vi "MotorsGoToLimits.vi"(11 "output cluster":T1) -> (0 "error out":errorcluster)   [LabVIEW 2015]
uses:
  Controls/LP Motor Thread Data.ctl
  Controls/LP Absolute Position Typedef.ctl
  Controls/LP Axis Enum Typedef.ctl
  MDrive Mode.ctl
  Get Parameter.ctl
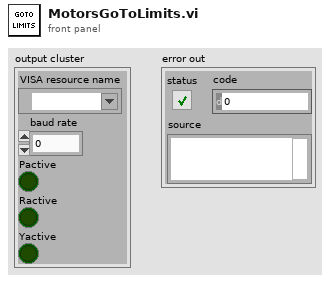
[diagram p1: front panel]
types:
  T1 = typedef "LP Motor Thread Data.ctl" = cluster{"VISA resource name":refnum<visa-resource-name>, "baud rate":u32, "Pactive":bool, "Ractive":bool, "Yactive":bool}
  T2 = typedef "LP Absolute Position Typedef.ctl" = cluster{"Axis":T3, "Position":dbl}
  T3 = typedef "LP Axis Enum Typedef.ctl" = enum16{"Pitch", "Roll", "Yaw"}
  T4 = typedef "Get Parameter.ctl" = enum16{"Acceleration (A)", "Baud Rate (BD)", "Busy Flag (BY)", "Counter 1 (C1)", "Counter 2 (C2)", "Check Sum Enable (CK)", "Clock Mode (CM)", "Clock Mode Ratio (CR)", "Clock Mode Out Step Width (CW)", "Deceleration (D)", "Digital Filtering, Input 1 (D1)", "Digital Filtering, Input 2 (D2)", "Digital Filtering, Input 3 (D3)", "Digital Filtering, Input 4 (D4)", "Digital Filtering, Input 5 (D5)", "Digital Filtering, Input 9 (D9)", "Digital Filtering, Input 10 (D10)", "Digital Filtering, Input 11 (D11)", "Digital Filtering, Input 12 (D12)", "Deadband (DB)", "Enable/Disable Drive (DE)", "Device Name (DN)", "End Program Execution (E)", "Encoder Function Enable (EE)", "Encoder Lines (EL)", "Error Flag (EF)", "Error Variable (ER)", "Echo Mode (EM)", "Escape (ES)", "Execute Program at Address (EX)", "Hold Current (HC)", "Hold Current Delay Time (HI)", "Input 1 (I1)", "Input 2 (I2)", "Input 3 (I3)", "Input 4 (I4)", "Input 5 Analog (I5)", "Input 6 Encoder Index (I6)", "Input 9 (I9)", "Input 10 (I10)", "Input 11 (I11)", "Input 12 (I12)", "Input Low Byte (1-4) (IL)", "Input High Byte (9-12) (IH)", "Inputs Total (1-4,9-12) (IN)", "Internal Temperature (IT)", "Jog Enable (JE)", "Limit Stop Mode (LM)", "MicroStepping Select (MS)", "Motor Settling Delay Time (MT)", "Moving Flag (MV)", "Output 1 (O1)", "Output 2 (O2)", "Output 3 (O3)", "Output 4 (O4)", "Output 9 (O9)", "Output 10 (O10)", "Output 11 (O11)", "Output 12 (O12)", "Output High Byte (9-12) (OH)", "Output Low Byte (1-4) (OL)", "Output Total (1-4 and 9-12) (OT)", "Position (P)", "Position Captured at Trip (PC)", "Position Maintenance (PM)", "Part Number (PN)", "Party Mode (PY)", "Register 1 (R1)", "Register 2 (R2)", "Register 3 (R3)", "Register 4 (R4)", "Run Current (RC)", "Serial Number (SN)", "Stall Flag (ST)", "Stall Factor (SF)", "Stall Mode Set (SM)", "User Variables (UV)", "Velocity (V)", "Velocity Changing Flag (VC)", "Velocity Initial (VI)", "Version, Firmware (VR)", "Velocity Maximum (VM)", "Read Input1", "Read Input2"}
  T5 = typedef "MDrive Mode.ctl" = enum16{"Normal Mode", "Party Mode"}
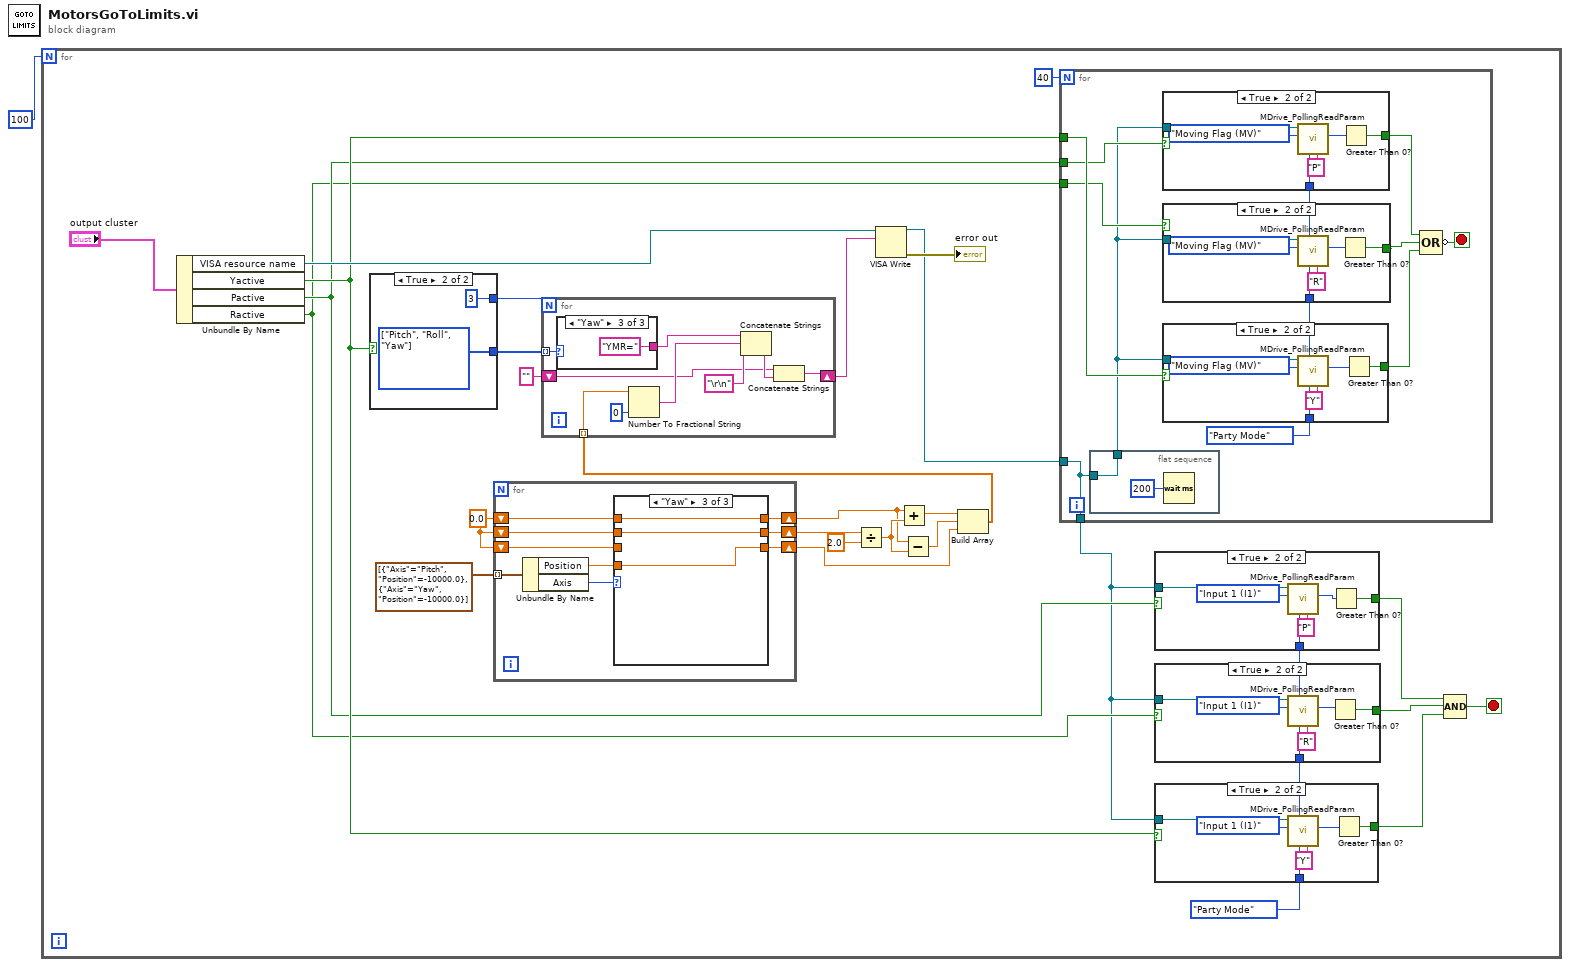
[diagram p0: block diagram]
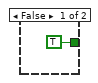
[diagram p2: hidden frame]
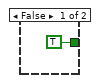
[diagram p3: hidden frame]
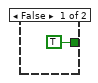
[diagram p4: hidden frame]
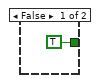
[diagram p5: hidden frame]
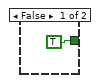
[diagram p6: hidden frame]
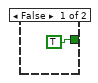
[diagram p7: hidden frame]
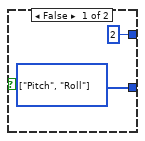
[diagram p8: hidden frame]
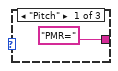
[diagram p9: hidden frame]
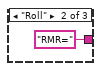
[diagram p10: hidden frame]
diagram:
  n1 = for {
    N: 100 -> [_]
    stop <- w7 stop-if-true
    w11 = MDrive_Mode."Party Mode" ("Mdrive Mode")
    w16 = 0.0 ("Position")
    n2 = Unbundle By Name("output cluster") -> ("VISA resource name"=w14:refnum<visa-resource-name>, "Yactive"=w5:bool, "Pactive"=w4:bool, "Ractive"=w3:bool)
    n3 = case shown="True" w5 {
      tunnel: [w85 w87] -> w22
      tunnel: [2 3] -> w28
      frame False {
        w85 = T3[] [enum."Pitch", enum."Roll"] items=["Pitch", "Roll", "Yaw"]
      }
      frame True {
        w87 = T3[] [enum."Pitch", enum."Roll", enum."Yaw"] items=["Pitch", "Roll", "Yaw"]
      }
    }
    n4 = for {
      tunnel: T2[] [{"Axis"=enum."Pitch", "Position"=-10000.0}, {"Axis"=enum."Yaw", "Position"=-10000.0}] ("data") -> [w108] mode=indexing
      shift-right: [w104] -> w17
      shift-left: w16 -> [w102]
      shift-right: [w106] -> w19
      shift-left: w16 -> [w100]
      shift-right: [w103] -> w27
      shift-left: w16 -> [w101]
      n5 = Unbundle By Name(w108) -> ("Position"=w105:dbl, "Axis"=w107:T3)
      n6 = case shown="\"Yaw\"" w107 {
        tunnel: [w109 w114 w117] -> w106
        tunnel: w105 -> [w109 w112 w115]
        tunnel: [w111 w112 w116] -> w104
        tunnel: [w110 w113 w115] -> w103
        tunnel: w102 -> [w111 _ w116]
        tunnel: w101 -> [w110 w113 _]
        tunnel: w100 -> [_ w114 w117]
        frame "Pitch" {
        }
        frame "Roll" {
        }
        frame "Yaw" {
        }
      }
    }
    n7 = Divide(x=w17, y=2.0) -> (x/y=w20:dbl)
    n8 = Add(x=w19, y=w20) -> (x+y=w23:dbl)
    n9 = Subtract(x=w19, y=w20) -> (x-y=w24:dbl)
    n10 = Build Array(w23, w24, w27) -> (w25:dbl[])
    n11 = for {
      N: w28 -> [_]
      shift-right: [w91] -> w26
      shift-left: "" -> [w90]
      tunnel: w22 -> [w89] mode=indexing
      tunnel: w25 -> [w88] mode=indexing
      n12 = case shown="\"Yaw\"" w89 {
        tunnel: ["PMR=" "RMR=" "YMR="] -> w92
        frame "Pitch" {
        }
        frame "Roll" {
        }
        frame "Yaw" {
        }
      }
      n13 = Number To Fractional String(number=w88, precision (6)=i16 0) -> (F-format string=w94:string)  [unwired: 2 in]
      n14 = Concatenate Strings(w92, w94, "\r\n") -> (w96:string)
      n15 = Concatenate Strings(w90, w96) -> (w91:string)
    }
    n16 = VISA Write(VISA resource name=w14, write buffer=w26) -> (VISA resource name out=w12:refnum<visa-resource-name>, error out=→"error out":errorcluster)  [unwired: 1 in, 1 out]
    n17 = for {
      N: 40 -> [_]
      tunnel: w12 -> [w55]
      tunnel: w5 -> [w59]
      tunnel: w4 -> [w58]
      tunnel: w3 -> [w57]
      tunnel: [w55] -> w2
      stop <- w51 stop-if-true
      w60 = MDrive_Mode."Party Mode" ("Mdrive Mode")
      n18 = flat-sequence {
        tunnel: [w61] -> w56
        tunnel: w55 -> [w61]
        frame #0 {
          n19 = Wait (ms)(milliseconds to wait=u32 200) -> ()  [unwired: 1 out]
        }
      }
      n20 = case shown="True" w58 {
        tunnel: w56 -> [_ w82]
        tunnel: w60 -> [_ w80]
        tunnel: [TRUE w78] -> w54
        frame False {
        }
        frame True {
          n21 = call "MDrive_PollingReadParam.vi"("Device Name"="P", "Mdrive Mode"=w80, "Get Parameter"=Get_Parameter."Moving Flag (MV)", "VISA Refnum in"=w82) -> ("Value"=w79:i32)  [unwired: 4 in, 3 out]
          n22 = Greater Than 0?(x=w79) -> (x > 0?=w78:bool)
        }
      }
      n23 = case shown="True" w57 {
        tunnel: w56 -> [_ w75]
        tunnel: w60 -> [_ w73]
        tunnel: [TRUE w71] -> w53
        frame False {
        }
        frame True {
          n24 = call "MDrive_PollingReadParam.vi"("Device Name"="R", "Mdrive Mode"=w73, "Get Parameter"=Get_Parameter."Moving Flag (MV)", "VISA Refnum in"=w75) -> ("Value"=w72:i32)  [unwired: 4 in, 3 out]
          n25 = Greater Than 0?(x=w72) -> (x > 0?=w71:bool)
        }
      }
      n26 = case shown="True" w59 {
        tunnel: w56 -> [_ w68]
        tunnel: w60 -> [_ w66]
        tunnel: [TRUE w64] -> w52
        frame False {
        }
        frame True {
          n27 = call "MDrive_PollingReadParam.vi"("Device Name"="Y", "Mdrive Mode"=w66, "Get Parameter"=Get_Parameter."Moving Flag (MV)", "VISA Refnum in"=w68) -> ("Value"=w65:i32)  [unwired: 4 in, 3 out]
          n28 = Greater Than 0?(x=w65) -> (x > 0?=w64:bool)
        }
      }
      n29 = Compound Arithmetic op=OR(w54, w53, w52) -> (invert w51:bool)
    }
    n30 = case shown="True" w4 {
      tunnel: w2 -> [_ w49]
      tunnel: w11 -> [_ w47]
      tunnel: [TRUE w45] -> w10
      frame False {
      }
      frame True {
        n31 = call "MDrive_PollingReadParam.vi"("Device Name"="P", "Mdrive Mode"=w47, "Get Parameter"=Get_Parameter."Input 1 (I1)", "VISA Refnum in"=w49) -> ("Value"=w46:i32)  [unwired: 4 in, 3 out]
        n32 = Greater Than 0?(x=w46) -> (x > 0?=w45:bool)
      }
    }
    n33 = case shown="True" w3 {
      tunnel: w2 -> [_ w42]
      tunnel: w11 -> [_ w40]
      tunnel: [TRUE w38] -> w9
      frame False {
      }
      frame True {
        n34 = call "MDrive_PollingReadParam.vi"("Device Name"="R", "Mdrive Mode"=w40, "Get Parameter"=Get_Parameter."Input 1 (I1)", "VISA Refnum in"=w42) -> ("Value"=w39:i32)  [unwired: 4 in, 3 out]
        n35 = Greater Than 0?(x=w39) -> (x > 0?=w38:bool)
      }
    }
    n36 = case shown="True" w5 {
      tunnel: w2 -> [_ w35]
      tunnel: w11 -> [_ w33]
      tunnel: [TRUE w31] -> w8
      frame False {
      }
      frame True {
        n37 = call "MDrive_PollingReadParam.vi"("Device Name"="Y", "Mdrive Mode"=w33, "Get Parameter"=Get_Parameter."Input 1 (I1)", "VISA Refnum in"=w35) -> ("Value"=w32:i32)  [unwired: 4 in, 3 out]
        n38 = Greater Than 0?(x=w32) -> (x > 0?=w31:bool)
      }
    }
    n39 = Compound Arithmetic op=AND(w10, w9, w8) -> (w7:bool)
  }
